vi "VI Konfig FID.vi"() -> ()   [LabVIEW 2015]
uses:
  CalGas Aufschaltung/FGV CalGas Aktionen.ctl
  CalGas Aufschaltung/CalGas Aufschaltung.lvlib
  FT-IR/FT-IR.lvlib
  FT-IR/FGV FT-IR Gasliste Aktionen.ctl
  Allgemein/allgemeine Sub-VIs.lvlib
  Passwortverwaltung/Passwort.lvlib
  Passwortverwaltung/FGV Passwort Aktion.ctl
  Grafik/Grafik.lvlib
  Seiten/NDIR-PMA-FID/Komm AO2000/Aktionen Diagnosewerte.ctl
  Messdaten/Messdaten.lvlib
  Messdaten/Aktionen FGV Messdaten.ctl
  Seiten/ABB Kalibrieren/Komm AO2000/Uras26 Kalibrierung.ctl
  cRIO/PC/Kommunikation mit cRIO.lvlib
  cRIO/PC/Aktionen - Lesen, schreiben.ctl
  Analysator Definition/Analysator Definition.lvlib
  Analysator Definition/FGV Analysator Definition Aktionen.ctl
  Seiten/ABB Kalibrieren/Komm AO2000/Aktionen FID Kal Komponente.ctl
  Visualisierungs Elemente/Zahlen-Ausgabefeld.ctl
  Visualisierungs Elemente/Auswahlfeld.ctl
  Visualisierungs Elemente/Button.ctl
  CalGas Aufschaltung/Aufschaltung CalGas_ANZEIGE.ctl
  ABB Kalibrieren/Komm AO2000/FID Kal Komponente.ctl
panel:
  in  "FID Kal Komponente":T1
  in  "Messbereich O2":T2 items=["0-500"=1, "0-2500"=2, "0-10000"=3]
  in  "Messbereich HC":T2 items=["0-500"=1, "0-2500"=2, "0-10000"=3]
  in  "Status AO":T3
  out "Flow PMA":T4 format="%.1f"
  in  "PMA Endpunkt":T3
  in  "PMA 0-Punkt":T3
  out "O2":string
  out "Mwert 2":sgl format="%.3f"
  out "PMwert 2":sgl format="%.3f"
  out "Wert 2":T4 caption="Konzentration" format="%.3f"
  in  "Kalibrierdaten":T3
  out "Mwert":sgl format="%.3f"
  out "PMwert":sgl format="%.3f"
  out "Wert":T4 caption="Konzentration" format="%.1f"
  out "Flow":T4 format="%.1f"
  out "Ausgang":T4 format="%.1f"
  out "Eingang":T4 format="%.1f"
  out "Druck H2He":T4 format="%.1f"
  out "Druck Brennluft":T4 format="%.1f"
  out "Temp Flamme":T4 format="%.1f"
  out "Temp Detektor":T4 format="%.1f"
  out "CH4":string
  in  "CH4 Endpunkt":T3
  in  "CH4 0-Punkt":T3
  out "Graph 1":waveform(dbl)[](graph)
  in  "Aufschaltung CalGas":T5 {"Analysator" items=["FT-IR", "FID", "PMA"]; "Aufschaltpunkt" items=["über Filterblock", "Analysator direkt", "über Gasteiler"]; "Kalibriergas" items=["Stickstoff", "", "", "", "", "", "", "", "", "", "", "", ""]}
  out "Graph 2":waveform(dbl)[](graph)
  # "Konfiguration FID / PMA"
  # "FID"
  # "PMA"
  # "±"
  # "±"
  # "Temperatur Detektor:"
  # "°C"
  # "Druck Eingang:"
  # "hPa"
  # "Temperatur Flamme:"
  # "°C"
  # "Druck Ausgang:"
  # "hPa"
  # "Druck Brennluft:"
  # "hPa"
  # "Flow:"
  # "l/h"
  # "Flow:"
  # "l/min"
  # "Druck Brenngas:"
  # "hPa"
  # "FID Kalibrieren mit:"
  # "Aufschaltung Kalibriergas"
  # "Kalibriergas"
  # "Aufschaltpunkt"
  # "Analysator"
  # "x"
  # "x"
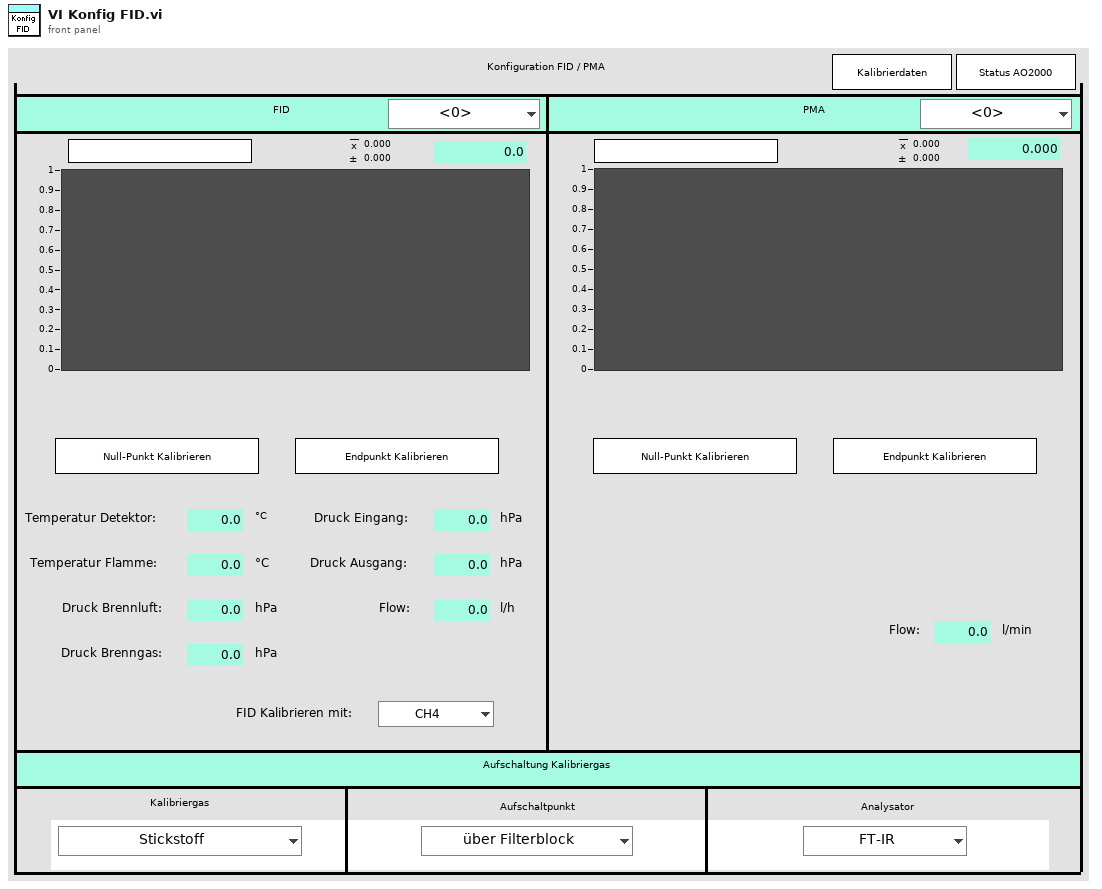
[diagram p1: front panel]
types:
  T1 = typedef "ABB Kalibrieren.lvlib/EL3000.lvlib/FID Kal Komponente.ctl" = enum16{"CH4", "C3H8"}
  T2 = typedef "Auswahlfeld.ctl" = u16
  T3 = typedef "Button.ctl" = bool
  T4 = typedef "Zahlen-Ausgabefeld.ctl" = sgl
  T5 = typedef "CalGas Aufschaltung.lvlib/Aufschaltung CalGas_ANZEIGE.ctl" = cluster{"Kalibriergas":T2, "Aufschaltpunkt":T2, "Analysator":T2}
  T6 = typedef "ABB Kalibrieren.lvlib/EL3000.lvlib/Aktionen FID Kal Komponente.ctl" = enum16{"lesen", "setzen", "laden", "speichern"}
  T7 = typedef "CalGas Aufschaltung.lvlib/FGV CalGas Aktionen.ctl" = enum16{"lesen", "Def.CalGas", "Aufschaltung CalGas", "laden", "speichern", "KAL extrahieren"}
  T8 = typedef "FT-IR.lvlib/FGV FT-IR Gasliste Aktionen.ctl" = enum16{"lesen", "Gasliste FT-IR", "Gasliste ausgelesen", "laden", "speichern", "löschen"}
  T9 = typedef "String - Ausgabefeld.ctl" = string
  T10 = typedef "CalGas Aufschaltung.lvlib/Aufschaltung CalGas.ctl" = cluster{"Kalibriergas":T2, "Aufschaltpunkt":T11, "Analysator":T12}
  T11 = typedef "CalGas Aufschaltung.lvlib/Auswahl Aufschaltpunkt.ctl" = enum16{"über Filterblock", "Analysator direkt", "über PNS"}
  T12 = typedef "CalGas Aufschaltung.lvlib/Auswahl Analysator.ctl" = enum16{"FT-IR", "PMA", "FID"}
  T13 = typedef "CalGas Aufschaltung.lvlib/Definition CalGas Anzeige.ctl" = cluster{"Namen":T14, "Werte":T16, "Werte 2":T16, "Einheit":T18, "Messbereiche":T19}
  T14 = typedef "CalGas Aufschaltung.lvlib/CalGas-Namen.ctl" = cluster{"Name":T15, "Name 2":T15, "Name 3":T15, "Name 4":T15, "Name 5":T15, "Name 6":T15, "Name 7":T15, "Name 8":T15, "Name 9":T15, "Name 10":T15, "Name 11":T15, "Name 12":T15}
  T15 = typedef "String - Eingabefeld.ctl" = string
  T16 = typedef "CalGas Aufschaltung.lvlib/CalGas-Werte.ctl" = cluster{"Konzentration 1":T17, "Konzentration 2":T17, "Konzentration 3":T17, "Konzentration 4":T17, "Konzentration 5":T17, "Konzentration 6":T17, "Konzentration 7":T17, "Konzentration 8":T17, "Konzentration 9":T17, "Konzentration 10":T17, "Konzentration 11":T17, "Konzentration 12":T17}
  T17 = typedef "Zahlen-Eingabefeld.ctl" = sgl
  T18 = typedef "CalGas Aufschaltung.lvlib/CalGas-Einheit.ctl" = cluster{"Einheit 1":T2, "Einheit 2":T2, "Einheit 3":T2, "Einheit 4":T2, "Einheit 5":T2, "Einheit 6":T2, "Einheit 7":T2, "Einheit 8":T2, "Einheit 9":T2, "Einheit 10":T2, "Einheit 11":T2, "Einheit 12":T2}
  T19 = typedef "CalGas Aufschaltung.lvlib/CalGas-Messbereiche.ctl" = cluster{"Messbereich 1":T2, "Messbereich 2":T2, "Messbereich 3":T2, "Messbereich 4":T2, "Messbereich 5":T2, "Messbereich 6":T2, "Messbereich 7":T2, "Messbereich 8":T2, "Messbereich 9":T2, "Messbereich 10":T2, "Messbereich 11":T2, "Messbereich 12":T2}
  T20 = typedef "Kommunikation mit cRIO.lvlib/Aktionen - Lesen, schreiben.ctl" = enum16{"lesen", "schreiben"}
  T21 = typedef "Messdaten.lvlib/Aktionen FGV Messdaten.ctl" = enum16{"lesen", "schreiben", "löschen", "Mittelwerte", "Komponente"}
  T22 = typedef "ABB Kalibrieren.lvlib/KOMM AO2000.lvlib/Aktionen Diagnosewerte.ctl" = enum16{"lesen", "schreiben"}
  T23 = typedef "Passwort.lvlib/FGV Passwort Aktion.ctl" = enum16{"prüfen", "setzen", "Initialisieren", "PW speichern", "lesen", "PW Änderung"}
  T24 = typedef "ABB Kalibrieren.lvlib/EL3000.lvlib/Typdefinitionen.lvlib/Uras26 Kalibrierung.ctl" = enum16{"Nullpunkt CO lo", "Nullpunkt CO hi", "Nullpunkt CO2 lo", "Nullpunkt CO2 hi", "Nullpunkt  HC", "Nullpunkt O2", "Endwert CO lo", "Endwert COhi", "Endwert CO2 lo", "Endwert CO2 hi", "Endwert HC", "Endwert O2"}
  T25 = typedef "Analysator Definition.lvlib/FGV Analysator Definition Aktionen.ctl" = enum16{"lesen", "MB setzen", "MB KAL setzen", "laden"}
  T26 = typedef "ABB Kalibrieren.lvlib/KOMM AO2000.lvlib/Typdefinitionen.lvlib/AO2000 - Diagnosewerte.ctl" = cluster{"FID - Temp Messzelle":sgl, "FID - Temperatur Flamme":sgl, "FID - Druck Brennluft":sgl, "FID - Druck H2":sgl, "FID - Druck Eingang":sgl, "FID - Druck Ausgang":sgl, "FID - Flow":sgl}
  T27 = cluster{"AI0: Durchfluss FT-IR":sgl, "AI1: Druck Ausgang":sgl, "AI2: Abs.Druck Kalt":sgl, "AI3: Druck FT-IR":sgl, "AI4: Druck CalGas":sgl, "AI5: Taupunktsensor":sgl, "AI6: Flowsensor PMA":sgl, "AI7: Druck CG PMA":sgl, "Rohwert Durchfluss FT-IR":sgl, "Rohwert Druck Ausgang":sgl, "Rohwert Druck Kalt":sgl, "Rohwert Durck FTIR":sgl, "Rohwert Druck CG":sgl, "Rohwert Taupunktsensor":sgl, "Rohwert Flow PMA":sgl, "Rohwert Druck CG PMA":sgl, "Schaltschrank":sgl, "Filter":sgl, "Pumpe":sgl, "HL BMP zu Filter":sgl, "HL zu FT-IR":sgl, "HL Extern SP1":sgl, "HL zu FID":sgl, "Reserve":sgl, "Reserve":sgl, "Reserve":sgl, "Reserve":sgl, "Reserve":sgl, "FT-IR":sgl, "Kühler FT-IR":sgl, "Gaskühler":sgl, "Reserve":sgl}
  T28 = cluster{"[0]":waveform(dbl), "[1]":waveform(dbl)}
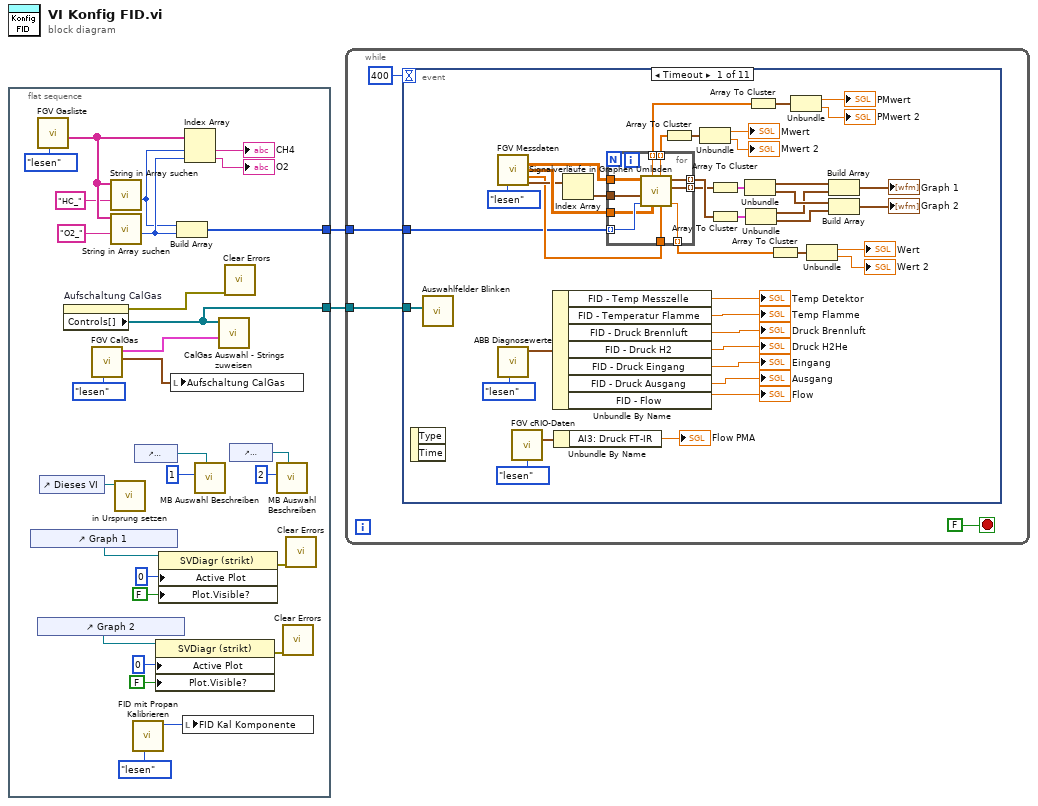
[diagram p0: block diagram]
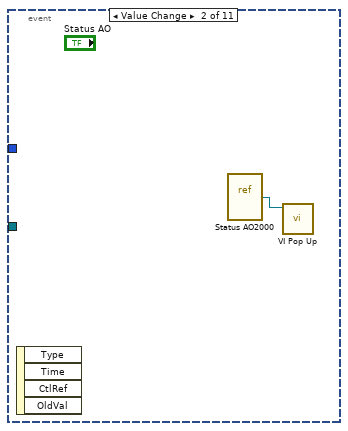
[diagram p2: hidden frame]
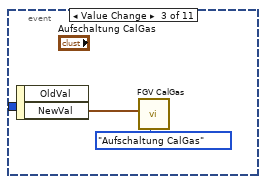
[diagram p3: hidden frame]
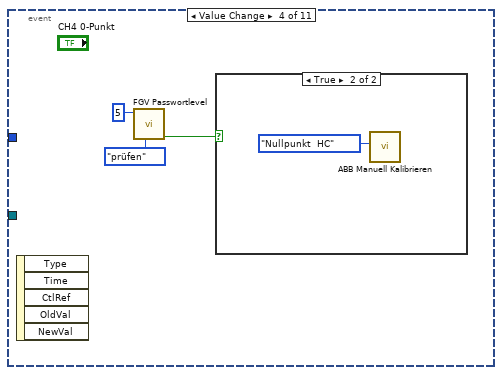
[diagram p4: hidden frame]
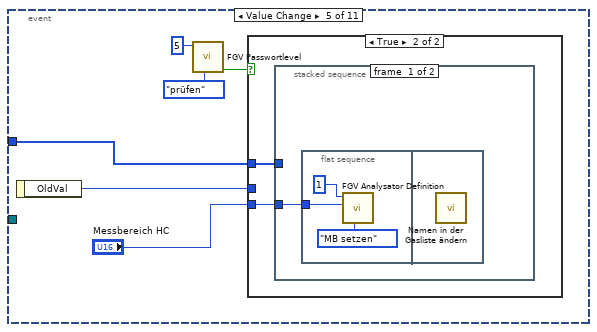
[diagram p6: hidden frame]
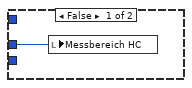
[diagram p7: hidden frame]
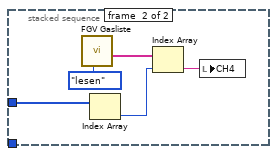
[diagram p8: hidden frame]
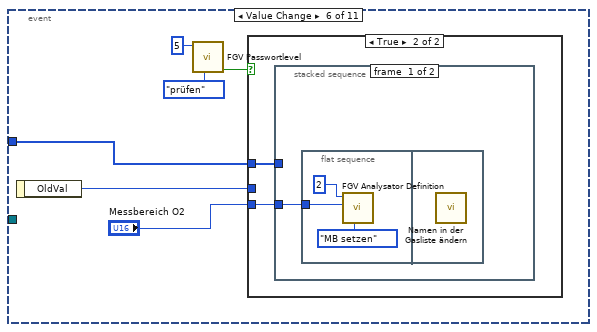
[diagram p9: hidden frame]
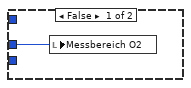
[diagram p10: hidden frame]
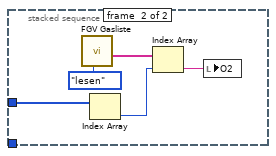
[diagram p11: hidden frame]
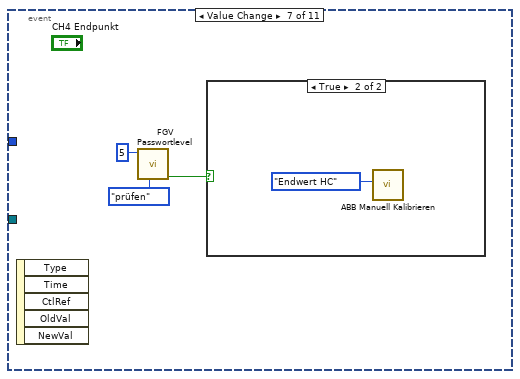
[diagram p12: hidden frame]
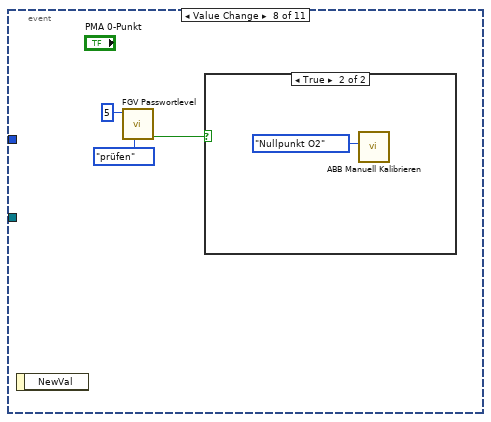
[diagram p14: hidden frame]
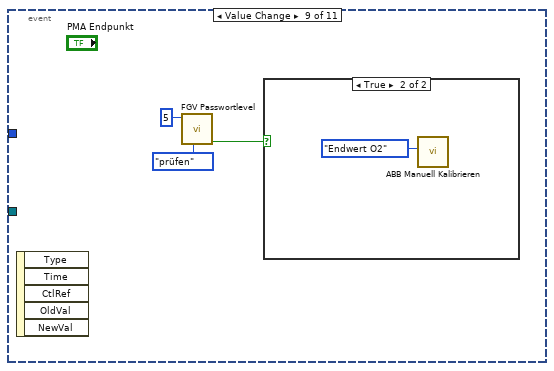
[diagram p16: hidden frame]
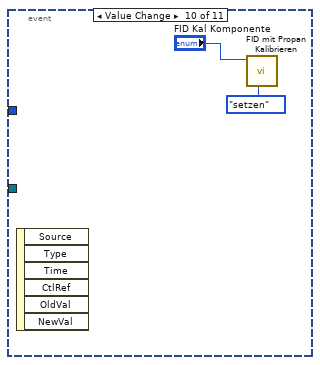
[diagram p18: hidden frame]
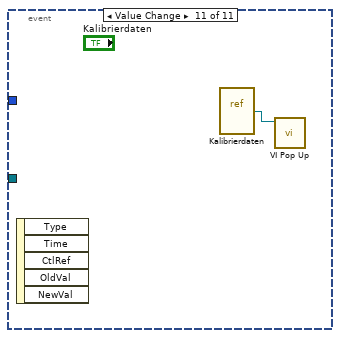
[diagram p19: hidden frame]
diagram:
  n1 = flat-sequence {
    tunnel: [w23] -> w2
    tunnel: [w22] -> w1
    frame #0 {
      n2 = control-ref of="Graph 1"() -> (w6:refnum<vi>)
      n3 = call "FGV Gasliste.vi"("Aktionen"=FGV_FT-IR_Gasliste_Aktionen."lesen") -> ("Aktuelle Gasliste gesamt"=w29:T9[])  [unwired: 8 in, 2 out]
      n4 = control-ref of="Graph 2"() -> (w5:refnum<vi>)
      n5 = control-ref of="Dieses VI"() -> (w13:refnum<vi>)
      n6 = property on="Aufschaltung CalGas" class="Cluster (strikt)"() -> (error out=w18:errorcluster, "Controls[]"=w22:refnum<vi>[])  [unwired: 2 in, 1 out]
      n7 = call "FGV CalGas.vi"("Aktionen"=FGV_CalGas_Aktionen."lesen") -> ("Aufschaltung CalGas"=w20:T10, "Def.CalGas"=w19:T13)  [unwired: 7 in, 2 out]
      n8 = call "String in Array suchen.vi"("Nach String/Zeichen suchen (-)"="HC_" ("DataSocket:URL"), "String-Array"=w29) -> ("Index"=w27:i32)  [unwired: 8 in, 1 out]
      n9 = call "String in Array suchen.vi"("Nach String/Zeichen suchen (-)"="O2_" ("DataSocket:URL"), "String-Array"=w29) -> ("Index"=w28:i32)  [unwired: 8 in, 1 out]
      n10 = call "in Ursprung setzen.vi"("VI Referenz"=w13) -> ()  [unwired: 11 in]
      n11 = call "FID mit Propan Kalibrieren.vi"("Aktionen"=Aktionen_FID_Kal_Komponente."lesen") -> ("FID Kal Komponente"=w4:T1)  [unwired: 9 in, 1 out]
      n12 = control-ref of="Messbereich HC"() -> (w17:refnum<vi>)
      n13 = property class="SVDiagr (strikt)"(reference=w5, "Active Plot"=u32 0 ("Aktiver Plot"), "Plot.Visible?"=FALSE ("Plot.Sichtbar")) -> (error out=w7:errorcluster)  [unwired: 1 in, 1 out]
      n14 = property class="SVDiagr (strikt)"(reference=w6, "Active Plot"=u32 0 ("Aktiver Plot"), "Plot.Visible?"=FALSE ("Plot.Sichtbar")) -> (error out=w12:errorcluster)  [unwired: 1 in, 1 out]
      n15 = local write "Aufschaltung CalGas"(w20) -> ()
      n16 = Build Array(w27, w28) -> (w23:i32[])
      n17 = local write "FID Kal Komponente"(w4) -> ()
      n18 = Index Array(array=w29, index #1=w27, index #2=w28) -> (element #1=→"CH4":T9, element #2=→"O2":T9)
      n19 = call "MB Auswahl Beschreiben.vi"("Auswahl Referenz"=w17, "Komponente"=1) -> ()  [unwired: 10 in]
      n20 = call "CalGas Auswahl - Strings zuweisen.vi"("Def.CalGas"=w19, "Aufschaltung CalGas"=w22) -> ()  [unwired: 10 in]
      n21 = call <vilib>:"Clear Errors.vi"("error in (no error)"=w18) -> ()  [unwired: 5 in, 2 out]
      n22 = control-ref of="Messbereich O2"() -> (w15:refnum<vi>)
      n23 = call "MB Auswahl Beschreiben.vi"("Auswahl Referenz"=w15, "Komponente"=2) -> ()  [unwired: 10 in]
      n24 = call <vilib>:"Clear Errors.vi"("error in (no error)"=w7) -> ()  [unwired: 5 in, 2 out]
      n25 = call <vilib>:"Clear Errors.vi"("error in (no error)"=w12) -> ()  [unwired: 5 in, 2 out]
    }
  }
  n26 = while {
    tunnel: w2 -> [w33]
    tunnel: w1 -> [w32]
    stop <- FALSE stop-if-true
    n27 = event shown="[0] Timeout" {
      selector: _ -> [_ _ _ _ _ _ _ _ _ _ _]
      dyn-events: _ -> [_ _ _ _ _ _ _ _ _ _ _]
      timeout: 400 -> [_ _ _ _ _ _ _ _ _ _ _]
      tunnel: w33 -> [w40 _ _ _ w97 w115 _ _ _ _ _]
      tunnel: w32 -> [w39 _ _ _ _ _ _ _ _ _ _]
      event Timeout {
        n28 = event-data() -> ()  [unwired: 1 in, 2 out]
        n29 = call "Auswahlfelder Blinken.vi"("Controls[]"=w39) -> ()  [unwired: 11 in]
        n30 = call "FGV Messdaten.vi"("Aktionen"=Aktionen_FGV_Messdaten."lesen") -> ("Messdaten"=w59:sgl[][], "Mittelwertdaten"=w60:sgl[][], "Deviation"=w55:sgl[], "Zeitstempeln"=w57:timestamp[])  [unwired: 8 in, 3 out]
        n31 = call "ABB Diagnosewerte.vi"("Aktion"=Aktionen_Diagnosewerte."lesen") -> ("AO2000 Diagnosewerte"=w69:T26)  [unwired: 8 in, 2 out]
        n32 = call "FGV cRIO-Daten.vi"("Aktion"=Aktionen_-_Lesen,_schreiben."lesen") -> ("Analog Input"=w37:T27)  [unwired: 6 in, 8 out]
        n33 = Unbundle By Name(w69) -> ("FID - Temp Messzelle"=→"Temp Detektor":sgl, "FID - Temperatur Flamme"=→"Temp Flamme":sgl, "FID - Druck Brennluft"=→"Druck Brennluft":sgl, "FID - Druck H2"=→"Druck H2He":sgl, "FID - Druck Eingang"=→"Eingang":sgl, "FID - Druck Ausgang"=→"Ausgang":sgl, "FID - Flow"=→"Flow":sgl)
        n34 = Unbundle By Name(w37) -> ("AI3: Druck FT-IR"=→"Flow PMA":sgl)
        n35 = Index Array(array=w57) -> (element=w56:timestamp)  [unwired: 1 in]
        n36 = for {
          tunnel: w40 -> [w87] mode=indexing
          tunnel: w59 -> [w86]
          tunnel: w56 -> [w85]
          tunnel: w60 -> [w84]
          tunnel: w55 -> [w83]
          tunnel: [w82] -> w54 mode=indexing
          tunnel: [w81] -> w51 mode=indexing
          tunnel: [w80] -> w52 mode=indexing
          tunnel: [w79] -> w42 mode=indexing
          tunnel: [w78] -> w41 mode=indexing
          n37 = call "Signalverläufe in Graphen Umladen.vi"("Deviation"=w83, "Mittelwertdaten"=w84, "Gas-Auswahl"=w87, "t0"=w85, "Werte"=w86) -> ("Konzentration"=w82:sgl, "Mittelwert"=w81:waveform(dbl), "Waveform"=w80:waveform(dbl), "aktuelle Mittelwert"=w79:sgl, "Deviation"=w78:sgl)  [unwired: 2 in]
        }
        n38 = Array To Cluster(array=w42) -> (cluster=w43:cluster{"[0]":sgl, "[1]":sgl})
        n39 = Unbundle(w43) -> ("[0]"=→"Mwert":sgl, "[1]"=→"Mwert 2":sgl)
        n40 = Array To Cluster(array=w51) -> (cluster=w49:T28)
        n41 = Array To Cluster(array=w52) -> (cluster=w50:T28)
        n42 = Unbundle(w49) -> ("[0]"=w48:waveform(dbl), "[1]"=w47:waveform(dbl))
        n43 = Unbundle(w50) -> ("[0]"=w46:waveform(dbl), "[1]"=w45:waveform(dbl))
        n44 = Array To Cluster(array=w41) -> (cluster=w44:cluster{"[0]":sgl, "[1]":sgl})
        n45 = Array To Cluster(array=w54) -> (cluster=w53:cluster{"[0]":sgl, "[1]":sgl})
        n46 = Unbundle(w44) -> ("[0]"=→"PMwert":sgl, "[1]"=→"PMwert 2":sgl)
        n47 = Unbundle(w53) -> ("[0]"=→"Wert":sgl, "[1]"=→"Wert 2":sgl)
        n48 = Build Array(w48, w46) -> (→"Graph 1":waveform(dbl)[])
        n49 = Build Array(w47, w45) -> (→"Graph 2":waveform(dbl)[])
      }
      event Value Change {
        n50 = event-data() -> ()  [unwired: 1 in, 4 out]
        n51 = vi-ref "Status AO2000.vi"() -> (w88:refnum<vi>)
        n52 = call "VI Pop Up.vi"("VI Referenz"=w88) -> ()  [unwired: 11 in]
      }
      event Value Change {
        n53 = event-data() -> ("NewVal"=w89:T5)  [unwired: 1 in, 1 out]
        n54 = call "FGV CalGas.vi"("Aktionen"=FGV_CalGas_Aktionen."Aufschaltung CalGas", "Aufschaltung CalGas"=w89) -> ()  [unwired: 6 in, 4 out]
      }
      event Value Change {
        n55 = event-data() -> ()  [unwired: 1 in, 5 out]
        n56 = call "FGV Passwortlevel.vi"("FGV Passwort Aktion"=FGV_Passwort_Aktion."prüfen", "geforderter Level"=i16 5) -> ("Freigabe"=w91:bool)  [unwired: 2 in, 7 out]
        n57 = case shown="True" w91 {
          frame False {
          }
          frame True {
            n58 = call "ABB Manuell Kalibrieren.vi"("Kalibrieren"=Uras26_Kalibrierung."Nullpunkt  HC") -> ()  [unwired: 11 in]
          }
        }
      }
      event Value Change {
        n59 = event-data() -> ("OldVal"=w96:T2)  [unwired: 1 in]
        n60 = call "FGV Passwortlevel.vi"("FGV Passwort Aktion"=FGV_Passwort_Aktion."prüfen", "geforderter Level"=i16 5) -> ("Freigabe"=w100:bool)  [unwired: 2 in, 7 out]
        n61 = case shown="True" w100 {
          tunnel: "Messbereich HC" -> [_ w103]
          tunnel: w96 -> [w101 _]
          tunnel: w97 -> [_ w102]
          frame False {
            n62 = local write "Messbereich HC"(w101) -> ()
          }
          frame True {
            n63 = stacked-sequence {
              tunnel: w103 -> [w104 _]
              tunnel: w102 -> [_ w109]
              frame #0 {
                n64 = flat-sequence {
                  tunnel: w104 -> [w105]
                  frame #0 {
                    n65 = call "FGV Analysator Definition.vi"("Aktionen"=FGV_Analysator_Definition_Aktionen."MB setzen", "Messbereich"=w105, "Komponente"=1) -> ()  [unwired: 6 in, 3 out]
                  }
                  frame #1 {
                    n66 = call "Namen in der Gasliste ändern.vi"() -> ()  [unwired: 12 in]
                  }
                }
              }
              frame #1 {
                n67 = call "FGV Gasliste.vi"("Aktionen"=FGV_FT-IR_Gasliste_Aktionen."lesen") -> ("Aktuelle Gasliste gesamt"=w112:T9[])  [unwired: 8 in, 2 out]
                n68 = Index Array(array=w109) -> (element=w108:i32)  [unwired: 1 in]
                n69 = Index Array(array=w112, index=w108) -> (element=w110:T9)
                n70 = local write "CH4"(w110) -> ()
              }
            }
          }
        }
      }
      event Value Change {
        n71 = event-data() -> ("OldVal"=w114:T2)  [unwired: 1 in]
        n72 = call "FGV Passwortlevel.vi"("FGV Passwort Aktion"=FGV_Passwort_Aktion."prüfen", "geforderter Level"=i16 5) -> ("Freigabe"=w118:bool)  [unwired: 2 in, 7 out]
        n73 = case shown="True" w118 {
          tunnel: "Messbereich O2" -> [_ w121]
          tunnel: w114 -> [w119 _]
          tunnel: w115 -> [_ w120]
          frame False {
            n74 = local write "Messbereich O2"(w119) -> ()
          }
          frame True {
            n75 = stacked-sequence {
              tunnel: w121 -> [w122 _]
              tunnel: w120 -> [_ w127]
              frame #0 {
                n76 = flat-sequence {
                  tunnel: w122 -> [w123]
                  frame #0 {
                    n77 = call "FGV Analysator Definition.vi"("Aktionen"=FGV_Analysator_Definition_Aktionen."MB setzen", "Messbereich"=w123, "Komponente"=2) -> ()  [unwired: 6 in, 3 out]
                  }
                  frame #1 {
                    n78 = call "Namen in der Gasliste ändern.vi"() -> ()  [unwired: 12 in]
                  }
                }
              }
              frame #1 {
                n79 = call "FGV Gasliste.vi"("Aktionen"=FGV_FT-IR_Gasliste_Aktionen."lesen") -> ("Aktuelle Gasliste gesamt"=w130:T9[])  [unwired: 8 in, 2 out]
                n80 = Index Array(array=w127) -> (element=w126:i32)  [unwired: 1 in]
                n81 = Index Array(array=w130, index=w126) -> (element=w128:T9)
                n82 = local write "O2"(w128) -> ()
              }
            }
          }
        }
      }
      event Value Change {
        n83 = event-data() -> ()  [unwired: 1 in, 5 out]
        n84 = call "FGV Passwortlevel.vi"("FGV Passwort Aktion"=FGV_Passwort_Aktion."prüfen", "geforderter Level"=i16 5) -> ("Freigabe"=w131:bool)  [unwired: 2 in, 7 out]
        n85 = case shown="True" w131 {
          frame False {
          }
          frame True {
            n86 = call "ABB Manuell Kalibrieren.vi"("Kalibrieren"=Uras26_Kalibrierung."Endwert HC") -> ()  [unwired: 11 in]
          }
        }
      }
      event Value Change {
        n87 = event-data() -> ()  [unwired: 1 in, 1 out]
        n88 = call "FGV Passwortlevel.vi"("FGV Passwort Aktion"=FGV_Passwort_Aktion."prüfen", "geforderter Level"=i16 5) -> ("Freigabe"=w135:bool)  [unwired: 2 in, 7 out]
        n89 = case shown="True" w135 {
          frame False {
          }
          frame True {
            n90 = call "ABB Manuell Kalibrieren.vi"("Kalibrieren"=Uras26_Kalibrierung."Nullpunkt O2") -> ()  [unwired: 11 in]
          }
        }
      }
      event Value Change {
        n91 = event-data() -> ()  [unwired: 1 in, 5 out]
        n92 = call "FGV Passwortlevel.vi"("FGV Passwort Aktion"=FGV_Passwort_Aktion."prüfen", "geforderter Level"=i16 5) -> ("Freigabe"=w141:bool)  [unwired: 2 in, 7 out]
        n93 = case shown="True" w141 {
          frame False {
          }
          frame True {
            n94 = call "ABB Manuell Kalibrieren.vi"("Kalibrieren"=Uras26_Kalibrierung."Endwert O2") -> ()  [unwired: 11 in]
          }
        }
      }
      event Value Change {
        n95 = event-data() -> ()  [unwired: 1 in, 6 out]
        n96 = call "FID mit Propan Kalibrieren.vi"("Aktionen"=Aktionen_FID_Kal_Komponente."setzen", "FID Kal Komponente 2"="FID Kal Komponente") -> ()  [unwired: 8 in, 2 out]
      }
      event Value Change {
        n97 = event-data() -> ()  [unwired: 1 in, 5 out]
        n98 = vi-ref "Kalibrierdaten.vi"() -> (w145:refnum<vi>)
        n99 = call "VI Pop Up.vi"("VI Referenz"=w145) -> ()  [unwired: 11 in]
      }
    }
  }
